vi "Door_polarity.vi"(0 "Strings in":string[](array[string])=["C:\\CuspControl\\GPIB and Network\\Cusp\\Dummyfile.txt", "6723"], 1 "Dubs in":dbl[](array[numeric])=[1.0]) -> ()   [LabVIEW 2018]
uses:
  <vilib>/DAQmx/write.llb/DAQmx Write (Analog DBL 1Chan 1Samp).vi
  <vilib>/DAQmx/create/channels.llb/DAQmx Create Channel (AO-Voltage-Basic).vi
  <vilib>/DAQmx/miscellaneous.llb/DAQmx Fill In Error Info.vi
panel:
  out "error out 2":errorcluster
  in  "milliseconds to drive relay":u32=10
  out "+/- out (V)":dbl=3.5
  in  "Polarity":bool=TRUE
  in  "|Coil voltage| (3.5 V)":dbl=3.5
  out "Elapsed time (ms)":u32=25
  in  "subvi":bool=TRUE
  out "error out":errorcluster
  in  "AO2 name":string="6723"
  in  "Relay lines":string[](array[string])=["/ao13", "/ao14"]
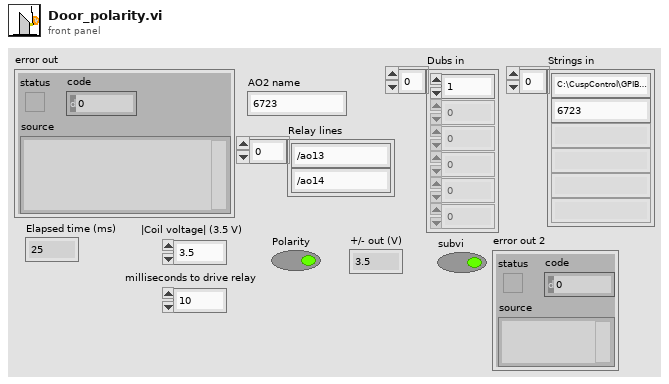
[diagram p1: front panel]
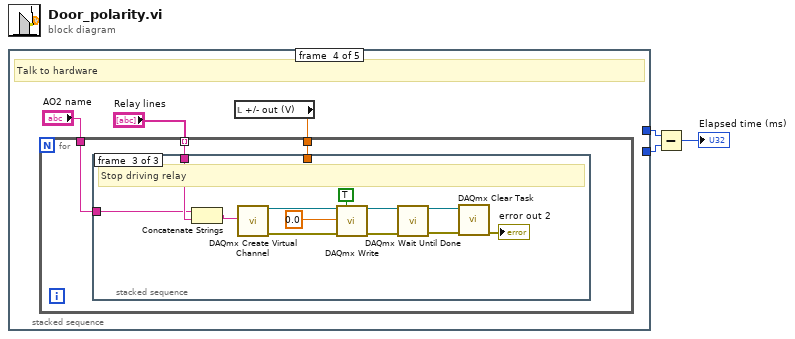
[diagram p0: block diagram]
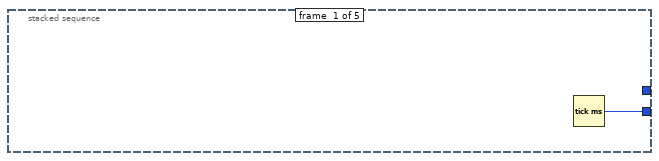
[diagram p2: hidden frame]
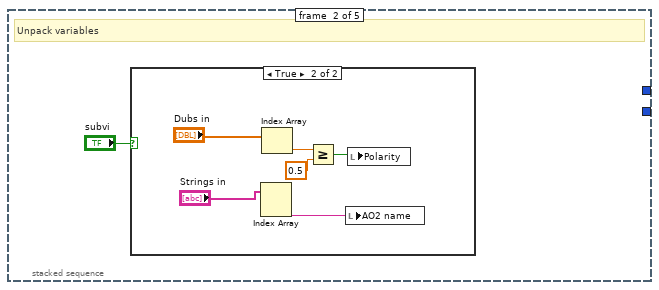
[diagram p3: hidden frame]
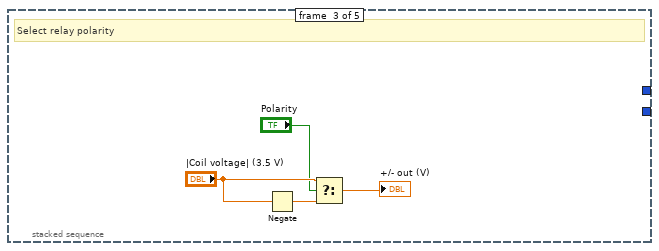
[diagram p5: hidden frame]
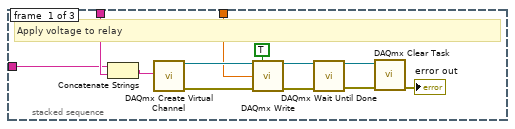
[diagram p6: hidden frame]
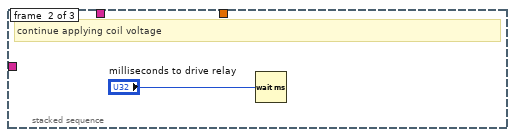
[diagram p7: hidden frame]
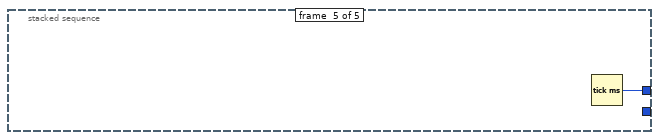
[diagram p8: hidden frame]
diagram:
  n1 = stacked-sequence {
    tunnel: [w4 _ _ _ _] -> w2
    tunnel: [_ _ _ _ w47] -> w3
    frame #0 {
      n2 = Tick Count (ms)() -> (millisecond timer value=w4:u32)
    }
    frame #1 {
      # "Unpack variables"
      n3 = case shown="True" "subvi" {
        frame False {
        }
        frame True {
          n4 = Index Array(array="Strings in") -> (element #2=w9:string)  [unwired: 2 in, 1 out]
          n5 = Index Array(array="Dubs in") -> (element=w8:dbl)  [unwired: 1 in]
          n6 = Greater Or Equal?(x=w8, y=0.5) -> (x >= y?=w6:bool)
          n7 = local write "AO2 name"(w9) -> ()
          n8 = local write "Polarity"(w6) -> ()
        }
      }
    }
    frame #2 {
      # "Select relay polarity"
      n9 = Negate(x="|Coil voltage| (3.5 V)") -> (-x=w15:dbl)
      n10 = Select(t="|Coil voltage| (3.5 V)", s="Polarity", f=w15) -> (s? t:f=→"+/- out (V)":dbl)
    }
    frame #3 {
      # "Talk to hardware"
      n11 = local read "+/- out (V)"() -> (w18:dbl)
      n12 = for {
        tunnel: w18 -> [w21]
        tunnel: "Relay lines" -> [w20] mode=indexing
        tunnel: "AO2 name" -> [w19]
        n13 = stacked-sequence {
          tunnel: w21 -> [w25 _ _]
          tunnel: w20 -> [w23 _ w38]
          tunnel: w19 -> [w22 _ w37]
          frame #0 {
            # "Apply voltage to relay"
            n14 = Concatenate Strings(w22, w23) -> (w29:string)
            n15 = call-poly <vilib>:"DAQmx Create Virtual Channel.vi"("physical channels"=w29) -> ("task out"=w27:refnum<k21>, "error out"=w26:errorcluster)  [unwired: 13 in]
            n16 = call-poly <vilib>:"DAQmx Write.vi"("task/channels in"=w27, "auto start"=TRUE, "data"=w25, "error in"=w26) -> ("task out"=w31:refnum<k21>, "error out"=w30:errorcluster)  [unwired: 9 in, 1 out]
            n17 = call <vilib>:"DAQmx Wait Until Done.vi"("task/channels in"=w31, "error in"=w30) -> ("task out"=w33:refnum<k21>, "error out"=w32:errorcluster)  [unwired: 12 in]
            n18 = call <vilib>:"DAQmx Clear Task.vi"("task in"=w33, "error in"=w32) -> ("error out"=→"error out":errorcluster)  [unwired: 13 in]
          }
          frame #1 {
            # "continue applying coil voltage"
            n19 = Wait (ms)(milliseconds to wait="milliseconds to drive relay") -> ()  [unwired: 1 out]
          }
          frame #2 {
            # "Stop driving relay"
            n20 = Concatenate Strings(w37, w38) -> (w42:string)
            n21 = call-poly <vilib>:"DAQmx Create Virtual Channel.vi"("physical channels"=w42) -> ("task out"=w41:refnum<k21>, "error out"=w40:errorcluster)  [unwired: 13 in]
            n22 = call-poly <vilib>:"DAQmx Write.vi"("task/channels in"=w41, "auto start"=TRUE, "data"=0.0, "error in"=w40) -> ("task out"=w44:refnum<k21>, "error out"=w43:errorcluster)  [unwired: 9 in, 1 out]
            n23 = call <vilib>:"DAQmx Wait Until Done.vi"("task/channels in"=w44, "error in"=w43) -> ("task out"=w46:refnum<k21>, "error out"=w45:errorcluster)  [unwired: 12 in]
            n24 = call <vilib>:"DAQmx Clear Task.vi"("task in"=w46, "error in"=w45) -> ("error out"=→"error out 2":errorcluster)  [unwired: 13 in]
          }
        }
      }
    }
    frame #4 {
      n25 = Tick Count (ms)() -> (millisecond timer value=w47:u32)
    }
  }
  n26 = Subtract(x=w3, y=w2) -> (x-y=→"Elapsed time (ms)":u32)
